vi "Get Boolean.vi"(8 "error in (no error)":errorcluster, 9 "Data Type (default value)":bool, 10 "Offset":i32, 11 "JSON":string) -> (0 "error out":errorcluster, 1 "Boolean":bool)   [LabVIEW 2013, in "JSONtext.lvlib"]
uses:
  JSONtext.lvlib
  String Subset.vi
  Advance past Number.vi
  Parsing Error.vi
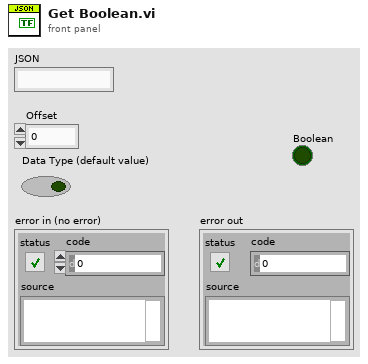
[diagram p1: front panel]
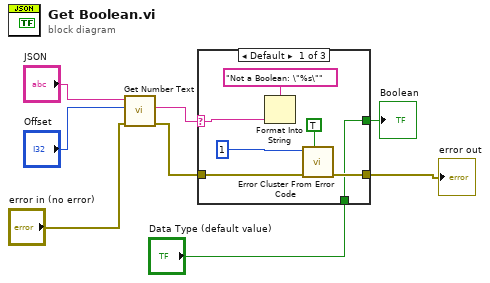
[diagram p0: block diagram]
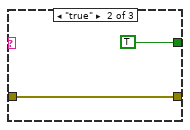
[diagram p2: hidden frame]
diagram:
  n1 = call "Get Number Text.vi"("error in (no error)"="error in (no error)", "Offset"="Offset", "JSON"="JSON") -> ("error out"=w2:errorcluster, "Number Text"=w5:string)  [unwired: 6 in, 1 out]
  n2 = case shown="Default" w5 {
    selector: w5 -> [w11 _ _]
    tunnel: [w9 TRUE _] -> w4
    tunnel: [w14 w16 w18] -> w3
    tunnel: w2 -> [w15 w16 w18]
    tunnel: "Data Type (default value)" -> [w9 _ _]
    frame Default {
      n3 = Format Into String(format string="Not a Boolean: \"%s\"", w11) -> ()  [unwired: 2 in, 2 out]
      n4 = call <vilib>:"Error Cluster From Error Code.vi"("show call chain? (False)"=TRUE, "error in (no error)"=w15, "error code (0)"=1) -> ("error out"=w14:errorcluster)  [unwired: 6 in]
    }
    frame "true" {
    }
    frame "false" {
    }
  }
  "error out" <- w3
  "Boolean" <- w4
